vi "Type Definitions(Exercise 5-3).vi"() -> ()   [LabVIEW 2014]
uses:
  Type Def Numeric.ctl
  Def Numeric.ctl
panel:
  in  "Type Def Numeric":u32
  in  "Type Def Numeric":T1
  in  "Strict Type Def Numeric":T2
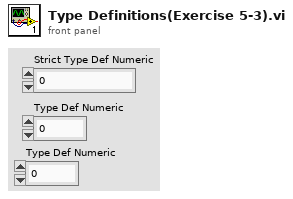
[diagram p1: front panel]
types:
  T1 = typedef "Def Numeric.ctl" = u32
  T2 = typedef "Type Def Numeric.ctl" = dbl
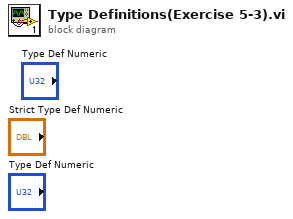
[diagram p0: block diagram]
diagram:
